vi "Thrust_vs_rpm.vi"() -> ()   [LabVIEW 2022 SP3]
uses:
  <vilib>/Analysis/NI_AALPro.lvlib
  <vilib>/DAQmx/create/channels.llb/DAQmx Create Channel (AI-Voltage-Basic).vi
  <resource>/objmgr/daqmx.rc
panel:
  out "Saved as":path caption="Filename Out"
  in  "Save file":bool=TRUE caption="Enable"
  out "Total thrust":dynamicdata(graph)
  out "Best Polynomial Fit":dbl[](array[numeric])
  out "Polynomial Coefficients":dbl[](array[numeric])
  in  "stop":bool
  out "Voltage":dynamicdata(graph)
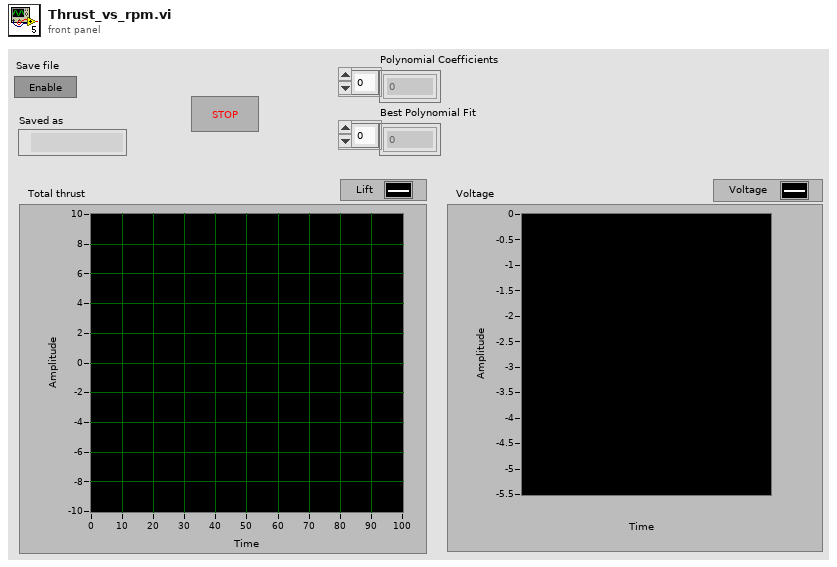
[diagram p1: front panel]
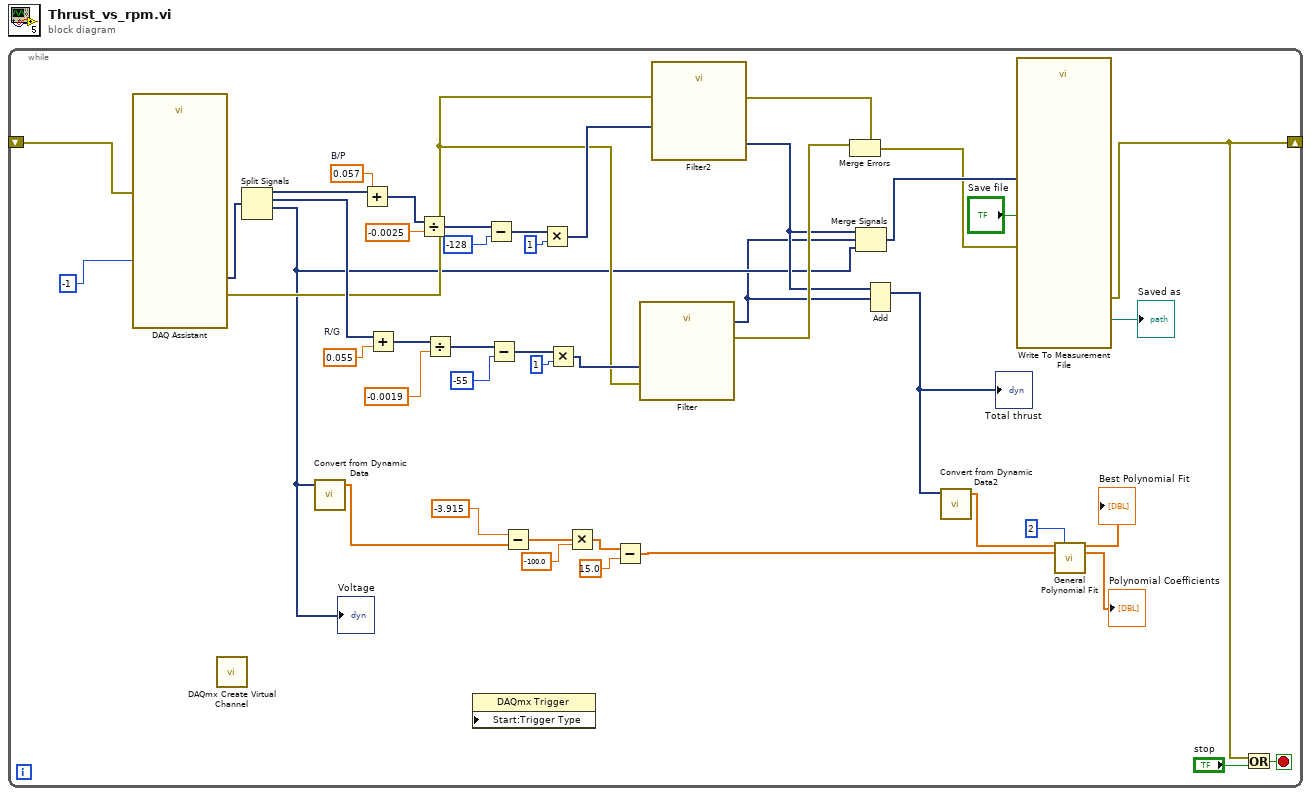
[diagram p0: block diagram]
diagram:
  n1 = while {
    shift-right: [w14] -> _
    shift-left: _ -> [w26]
    stop <- w8 stop-if-true
    w43 = 0.057  # B/P
    w44 = 0.055  # R/G
    n2 = call "DAQ Assistant"("timeout (s)"=-1, "error in"=w26) -> ("data"=w40:dynamicdata, "error out"=w17:errorcluster)  [unwired: 14 in, 2 out]
    n3 = call-poly <vilib>:"DAQmx Create Virtual Channel.vi"() -> ()  [unwired: 14 in, 2 out]
    n4 = Split Signals(w40) -> (w38:dynamicdata, w39:dynamicdata, w15:dynamicdata)  [unwired: 4 in, 1 out]
    "Voltage" <- w15
    n5 = call "Convert from Dynamic Data"("Dynamic Data Type"=w15) -> ("Array"=w13:dbl[])  [unwired: 3 in]
    n6 = Add(x=w38, y=w43) -> (x+y=w46:dynamicdata)
    n7 = Add(x=w39, y=w44) -> (x+y=w45:dynamicdata)
    n8 = Divide(x=w46, y=-0.0025) -> (x/y=w37:dynamicdata)
    n9 = Divide(x=w45, y=-0.0019) -> (x/y=w35:dynamicdata)
    n10 = property class="DAQmx Trigger" props=["Start:Trigger Type"]() -> ()  [unwired: 3 in, 2 out]
    n11 = Subtract(x=w37, y=-128) -> (x-y=w31:dynamicdata)
    n12 = Subtract(x=w35, y=-55) -> (x-y=w30:dynamicdata)
    n13 = Subtract(x=-3.915, y=w13) -> (x-y=w24:dbl[])
    n14 = Multiply(x=w31, y=1) -> (x*y=w23:dynamicdata)
    n15 = Multiply(x=w30, y=1) -> (x*y=w29:dynamicdata)
    n16 = Multiply(x=w24, y=-100.0) -> (x*y=w22:dbl[])
    n17 = Subtract(x=w22, y=15.0) -> (x-y=w9:dbl[])
    n18 = call "Filter"("error in (no error)"=w17, "Signal"=w29) -> ("error out"=w20:errorcluster, "Filtered Signal"=w3:dynamicdata)  [unwired: 8 in]
    n19 = call "Filter2"("error in (no error)"=w17, "Signal"=w23) -> ("error out"=w19:errorcluster, "Filtered Signal"=w16:dynamicdata)  [unwired: 8 in]
    n20 = Merge Errors(w20, w19) -> (w18:errorcluster)
    n21 = Merge Signals(w16, w3, w15) -> (w27:dynamicdata)
    n22 = Add(1:w3, 2:w16) -> (0:w4:dynamicdata)  [unwired: 1 in, 1 out]
    "Total thrust" <- w4
    n23 = call "Convert from Dynamic Data2"("Dynamic Data Type"=w4) -> ("Array"=w7:dbl[])  [unwired: 3 in]
    n24 = call "Write To Measurement File"("Signals"=w27, "Enable"="Save file", "error in (no error)"=w18) -> ("Filename Out"=→"Saved as":path, "error out"=w14:errorcluster)  [unwired: 14 in, 1 out]
    n25 = call <vilib>:"General Polynomial Fit.vi"("Y"=w7, "polynomial order"=2, "X"=w9) -> ("Best Polynomial Fit"=→"Best Polynomial Fit":dbl[], "Polynomial Coefficients"=→"Polynomial Coefficients":dbl[])  [unwired: 9 in, 2 out]
    n26 = Or(x=w14, y="stop") -> (x .or. y?=w8:bool)
  }
